vi "Add Parameter.vi"(4 "Ignored?":bool, 5 "Exception Value":string, 6 "Input?":bool, 7 "type":T1, 8 "error in (no error)":errorcluster, 9 "Description":string, 10 "Name":string, 11 "PyTool in":refnum<class "PyTool.lvclass">) -> (0 "error out":errorcluster, 3 "PyTool out":refnum<class "PyTool.lvclass">)   [LabVIEW 2025, in "Tools.lvlib" / "PyTool.lvclass"]
uses:
  PyTool.lvclass
  PyTool.lvclass/PyTool.ctl
  Datatypes.ctl
  Tools.lvlib
  Parameter.ctl
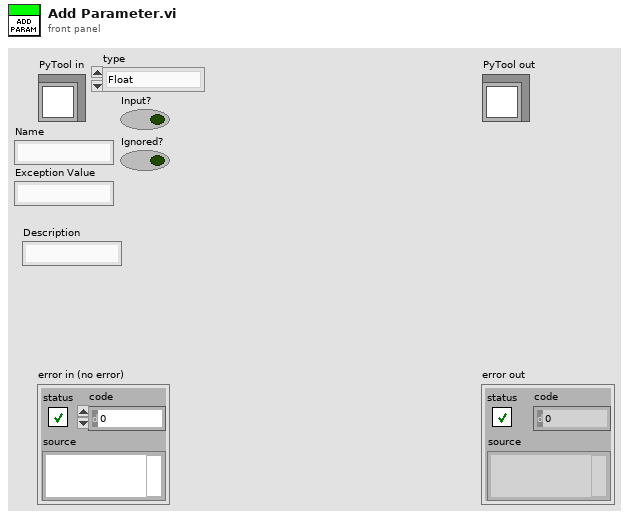
[diagram p1: front panel]
types:
  T1 = typedef "Tools.lvlib/Datatypes.ctl" = enum16{"Float", "Int", "String", "String Array", "Int Array", "Float Array", "Bool Array", "Bool", "Invalid"}
  T2 = typedef "Tools.lvlib/PyTool.lvclass/Parameter.ctl" = cluster{"Name":string, "type":T1, "Input?":bool, "Ignored?":bool, "Exception Value":string, "Description":string}
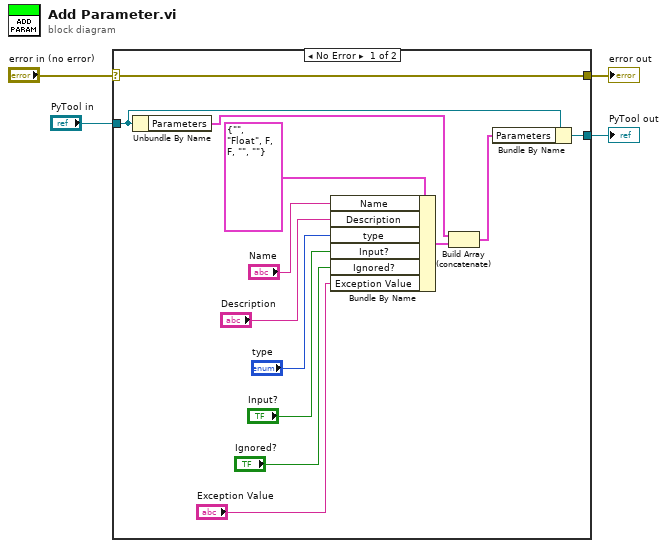
[diagram p0: block diagram]
diagram:
  n1 = case shown="No Error" "error in (no error)" {
    selector: "error in (no error)" -> [w17 w19]
    tunnel: [w17 w19] -> w3
    tunnel: [w16 w18] -> w1
    tunnel: "PyTool in" -> [w15 w18]
    frame No Error {
      n2 = Unbundle By Name(w15) -> ("Parameters"=w14:T2[])
      n3 = Bundle By Name(cluster=T2 {"Name"="", "type"=enum."Float", "Input?"=FALSE, "Ignored?"=FALSE, "Exception Value"="", "Description"=""} ("array"), "Name"="Name", "Description"="Description", "type"="type", "Input?"="Input?", "Ignored?"="Ignored?", "Exception Value"="Exception Value") -> (w11:T2)
      n4 = Build Array (concatenate)(w14, w11) -> (w13:T2[])
      n5 = Bundle By Name(cluster=w15, "Parameters"=w13) -> (w16:refnum<class "PyTool.lvclass">)
    }
    frame Error {
    }
  }
  "error out" <- w3
  "PyTool out" <- w1
